vi "AI-Motor_Close.vi"(8 "Error In":errorcluster) -> (0 "Error Out":errorcluster)   [LabVIEW 2019]
uses:
  <instrlib>/Dynamixel Motor/Public/Motor Operation/Low Level/Baud Setting.ctl
  Variable/Position.vi
  <instrlib>/Dynamixel Motor/Dynamixel Motor.lvlib
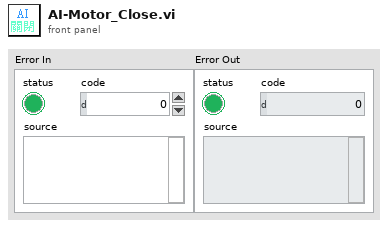
[diagram p1: front panel]
types:
  T1 = typedef "Dynamixel Motor.lvlib/Baud Setting.ctl" = u8
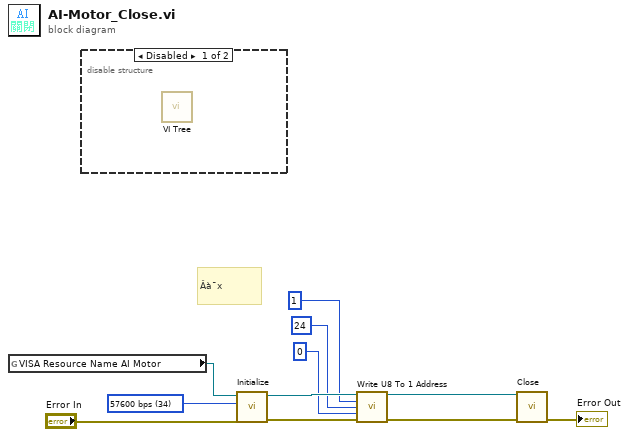
[diagram p0: block diagram]
diagram:
  w10 = T1 34 items=["1,000,000 bps"=1, "500,000 bps"=3, "400,000 bps"=4, "250,000 bps"=7, "200,000 bps"=9, "115200 bps"=16, "57600 bps"=34, "19200 bps"=103, "9600 bps"=207] ("Baud rate (57600 bps)")
  # "Âà¯x"
  n1 = global read "Position.vi" "VISA Resource Name AI Motor"() -> (w1:refnum<visa-resource-name>)
  n2 = disable-structure shown="Disabled" {
    frame Disabled {
      n3 = call <instrlib>:"VI Tree.vi"() -> ()  [unwired: 12 in]
    }
    frame Enabled {
    }
  }
  n4 = call <instrlib>:"Initialize.vi"("error in (no error)"="Error In", "Baud rate (57600 bps)"=w10, "VISA resource name"=w1) -> ("error out"=w8:errorcluster, "VISA resource name out"=w9:refnum<visa-resource-name>)  [unwired: 7 in]
  n5 = call <instrlib>:"Write U8 To 1 Address.vi"("VISA resource name"=w9, "Motor ID (0)"=u8 1, "Address number (0)"=u8 24, "Parameter (0)"=u8 0, "error in (no error)"=w8) -> ("VISA resource name out"=w3:refnum<visa-resource-name>, "error out"=w4:errorcluster)  [unwired: 9 in]
  n6 = call <instrlib>:"Close.vi"("error in (no error)"=w4, "VISA resource name"=w3) -> ("error out"=→"Error Out":errorcluster)  [unwired: 9 in]
